vi "Real Time Tracking System of a Colored object.vi"(0 "ROI Descriptor (Color Location 1)":T2={"Global Rectangle"=[20, 20, 1260, 700], "Contours"=[{"ID"=enum."External", "Type"=12, "Coordinates"=[20, 20, 1260, 700, 0]}]} {"Contours"."Type" items=["No Selection", "Point", "Line", "Rectangle", "Oval", "Polygon", "Freehand Region", "Annulus", "Unused2", "Unused3", "Broken Line", "Freehand Line", "Rotated Rectangle"]}, 1 "File Path (Color Location 1)":path=path "E:/engineering courses/my/Machine Vision LV/T.png", 2 "Minimum Match Score (Color Location 1)":sgl=800.0) -> (20 "Matches (Color Location 1)":T3(array[cluster]) {"Bounding Box"."y" format="%.2f"; "Bounding Box"."x" format="%.2f"; "Position"."y" format="%.2f"; "Position"."x" format="%.2f"; "Score" format="%.2f"; "Scale" format="%.2f"; "Angle" format="%.2f"}, 21 "Matches (calibrated) (Color Location 1)":T3(array[cluster]) {"Bounding Box"."y" format="%.2f"; "Bounding Box"."x" format="%.2f"; "Position"."y" format="%.2f"; "Position"."x" format="%.2f"; "Score" format="%.2f"; "Scale" format="%.2f"; "Angle" format="%.2f"}, 22 "Number of Matches (Color Location 1)":i32, 27 "error out":errorcluster)   [LabVIEW 2015]
uses:
  <vilib>/vision/NI_Vision_Development_Module.lvlib
  <resource>/objmgr/imaqdx.rc
  <vilib>/vision/driver/NI_Vision_Acquisition_Software.lvlib
panel:
  out "Image":T1(plugin-control)
  in  "Camera Name":refnum<k21> caption="IMAQdx Session"
  in  "Video Modes":i32(listbox)
  in  "Stop":bool
  out "Buffer Number":u32
  out "Frame Rate":dbl(knob) scale=0.0..100.0
  out "Image Out":T1(plugin-control)
  # "Machine vision application Developed \nBy Abdalrahman M. Amer \nMUST university @Egypt \nabdalrahman.m5959@gmail.com"
  # "Colored Object Tracking system"
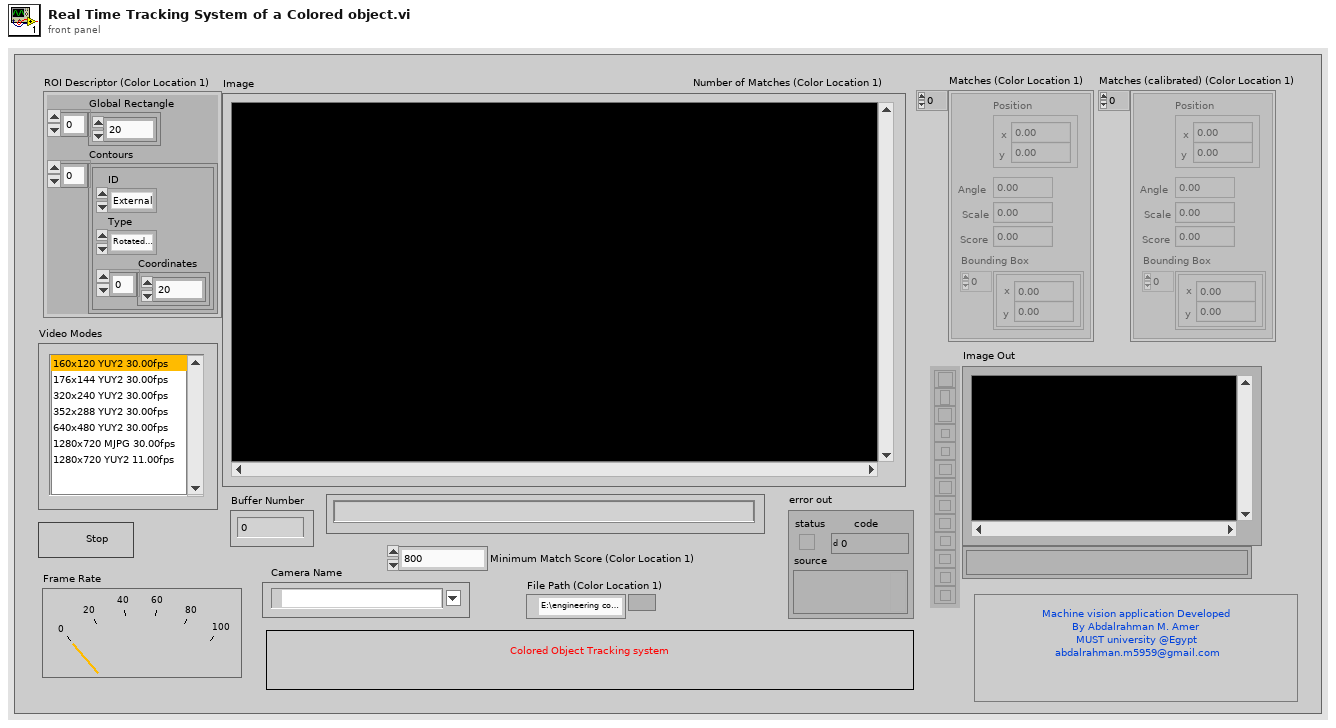
[diagram p1: front panel]
types:
  T1 = typedef "IMAQ Image.ctl" = refnum<image>
  T2 = cluster{"Global Rectangle":i32[], "Contours":cluster{"ID":enum32{"External", "Internal"}, "Type":u32, "Coordinates":i32[]}[]}
  T3 = cluster{"Position":cluster{"x":sgl, "y":sgl}, "Angle":sgl, "Scale":sgl, "Score":sgl, "Bounding Box":cluster{"x":sgl, "y":sgl}[]}[]
  T4 = typedef "IMAQdx.ctl" = refnum<k21>
  T5 = typedef "Image Type" = u32
  T6 = cluster{"Matches[0]":cluster{"Position":cluster{"x":sgl, "y":sgl}, "Angle":sgl, "Scale":sgl, "Score":sgl, "Bounding Box":cluster{"x":sgl, "y":sgl}[]}, "Matches[1]":cluster{"Position":cluster{"x":sgl, "y":sgl}, "Angle":sgl, "Scale":sgl, "Score":sgl, "Bounding Box":cluster{"x":sgl, "y":sgl}[]}, "Matches[2]":cluster{"Position":cluster{"x":sgl, "y":sgl}, "Angle":sgl, "Scale":sgl, "Score":sgl, "Bounding Box":cluster{"x":sgl, "y":sgl}[]}, "Matches[3]":cluster{"Position":cluster{"x":sgl, "y":sgl}, "Angle":sgl, "Scale":sgl, "Score":sgl, "Bounding Box":cluster{"x":sgl, "y":sgl}[]}, "Matches[4]":cluster{"Position":cluster{"x":sgl, "y":sgl}, "Angle":sgl, "Scale":sgl, "Score":sgl, "Bounding Box":cluster{"x":sgl, "y":sgl}[]}, "Matches[5]":cluster{"Position":cluster{"x":sgl, "y":sgl}, "Angle":sgl, "Scale":sgl, "Score":sgl, "Bounding Box":cluster{"x":sgl, "y":sgl}[]}, "Matches[6]":cluster{"Position":cluster{"x":sgl, "y":sgl}, "Angle":sgl, "Scale":sgl, "Score":sgl, "Bounding Box":cluster{"x":sgl, "y":sgl}[]}, "Matches[7]":cluster{"Position":cluster{"x":sgl, "y":sgl}, "Angle":sgl, "Scale":sgl, "Score":sgl, "Bounding Box":cluster{"x":sgl, "y":sgl}[]}, "Matches[8]":cluster{"Position":cluster{"x":sgl, "y":sgl}, "Angle":sgl, "Scale":sgl, "Score":sgl, "Bounding Box":cluster{"x":sgl, "y":sgl}[]}}
  T7 = cluster{"Position":cluster{"x":sgl, "y":sgl}, "Angle":sgl, "Scale":sgl, "Score":sgl, "Bounding Box":cluster{"x":sgl, "y":sgl}[]}
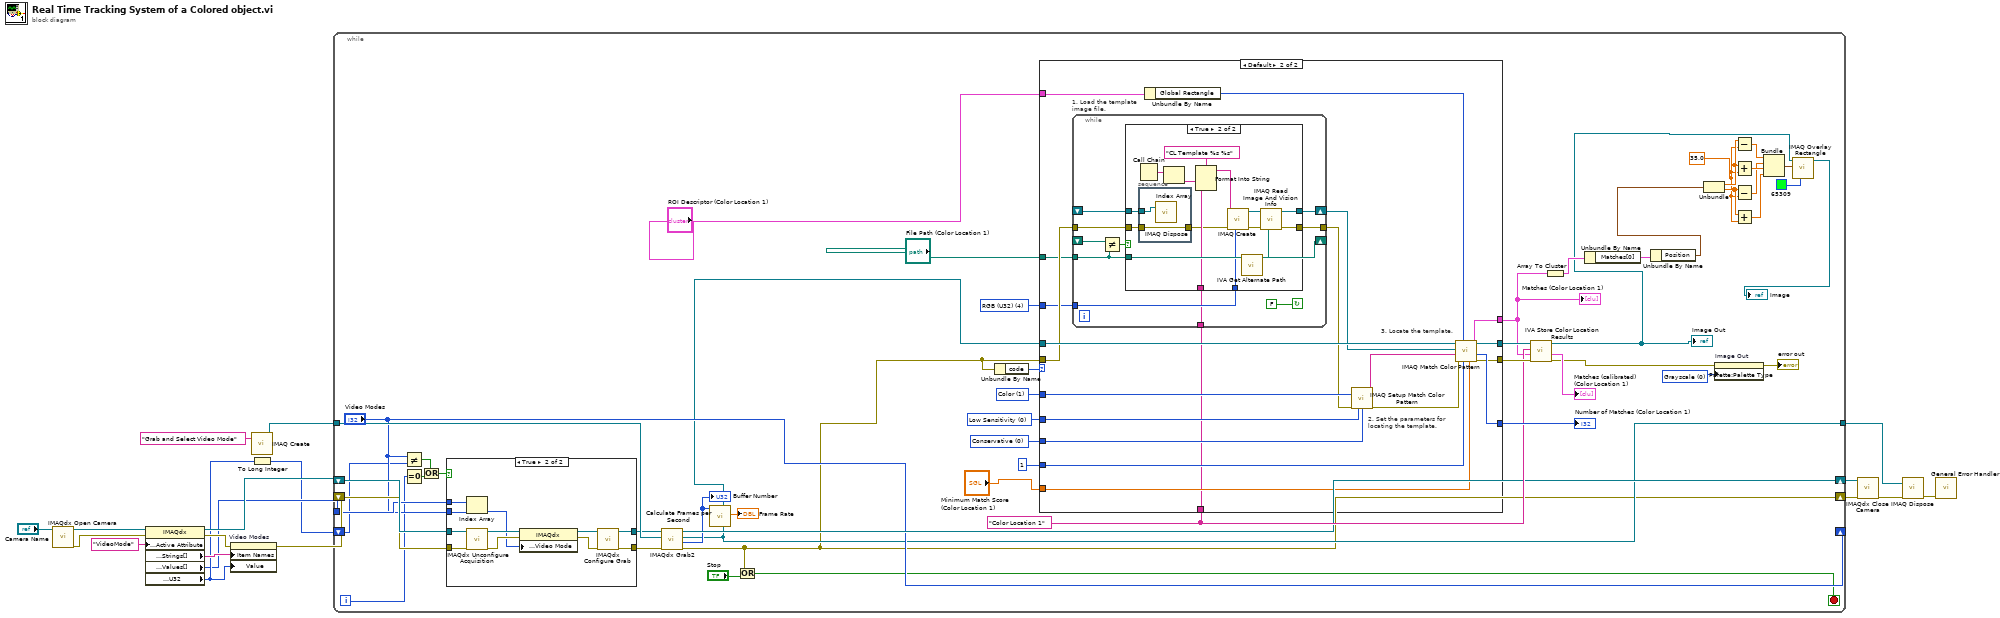
[diagram p0: block diagram]
diagram:
  n1 = call <vilib>:"IMAQdx Open Camera.vi"("Session In"="Camera Name") -> ("error out"=w11:errorcluster, "Session Out"=w13:T4)  [unwired: 2 in, 7 out]
  n2 = property class="IMAQdx"(reference=w13, error in=w11, "Camera Attributes:Active Attribute"="VideoMode" ("ActiveAttribute")) -> (reference out=w9:T4, error out=w10:errorcluster, "Camera Attributes:Enum:Strings[]"=w7:string[], "Camera Attributes:Enum:Values[]"=w2:u32[], "Camera Attributes:Value:U32"=w6:u32)
  n3 = property on="Video Modes" class="LstBox (strict)"(error in=w10, "Item Names"=w7, "Value"=w6) -> (error out=w8:errorcluster)  [unwired: 1 in, 1 out]
  n4 = call "IMAQ Create"("Image Name"="Grab and Select Video Mode") -> ("New Image"=w16:T1)  [unwired: 3 in, 2 out]
  n5 = To Long Integer(number=w6) -> (32bit integer=w1:i32)
  n6 = while {
    tunnel: w2 -> [w48]
    shift-right: [w51] -> w15
    shift-left: w9 -> [w50]
    shift-right: [w34] -> w18
    shift-left: w8 -> [w49]
    tunnel: w16 -> [w52]
    tunnel: [w35] -> w5
    shift-right: ["Video Modes"] -> _
    shift-left: w1 -> [w38]
    i -> [w36]
    stop <- w37 stop-if-true
    w20 = 35.0
    w53 = u32 0 items=["Grayscale", "Binary", "Gradient", "Rainbow", "Temperature", "User Defined", "Binary 16 Bit", "Gradient 16 Bit", "Rainbow 16 Bit", "Temperature 16 Bit", "User Defined 16 Bit"] ("Palette Type")
    w55 = "Color Location 1" ("Step Name")
    w62 = T5 4 items=["Grayscale (U8)", "Grayscale (I16)", "Grayscale (SGL)", "Complex (CSG)", "RGB (U32)", "HSL (U32)", "RGB (U64)"] ("Image Type")
    w64 = u32 0 items=["Conservative", "Balance", "Aggressive", "Very Aggressive"] ("Search Strategy")
    w65 = u32 0 items=["Low Sensitivity", "Medium Sensitivity", "High Sensitivity"] ("Color Sensitivity")
    w66 = u32 1 items=["Color and Shape", "Color", "Shape"] ("Match Feature Mode")
    n7 = Not Equal?(x="Video Modes", y=w38) -> (x != y?=w45:bool)
    n8 = Equal To 0?(x=w36) -> (x = 0?=w44:bool)
    n9 = Or(x=w45, y=w44) -> (x .or. y?=w46:bool)
    n10 = case shown="True" w46 {
      tunnel: w50 -> [w71 w80]
      tunnel: w49 -> [w70 w79]
      tunnel: [w71 w76] -> w42
      tunnel: [w70 w77] -> w43
      tunnel: w48 -> [_ w82]
      tunnel: "Video Modes" -> [_ w81]
      frame False {
      }
      frame True {
        n11 = Index Array(array=w82, index=w81) -> (element=w72:u32)
        n12 = call <vilib>:"IMAQdx Unconfigure Acquisition.vi"("error in"=w79, "Session In"=w80) -> ("error out"=w73:errorcluster, "Session Out"=w78:T4)  [unwired: 8 out]
        n13 = property class="IMAQdx"(reference=w78, error in=w73, "Acquisition Attributes:Video Mode"=w72) -> (reference out=w75:T4, error out=w74:errorcluster)
        n14 = call <vilib>:"IMAQdx Configure Grab.vi"("error in"=w74, "Session In"=w75) -> ("error out"=w77:errorcluster, "Session Out"=w76:T4)  [unwired: 1 in, 7 out]
      }
    }
    n15 = call <vilib>:"IMAQdx Grab2.vi"("error in"=w43, "Image In"=w52, "Session In"=w42) -> ("error out"=w34:errorcluster, "Buffer Number Out"=w40:u32, "Image Out"=w35:T1, "Session Out"=w51:T4)  [unwired: 5 in]
    "Buffer Number" <- w40
    n16 = call <vilib>:"Calculate Frames per Second.vi"("Buffer Number"=w40) -> ("Processed Frames/s"=→"Frame Rate":dbl)  [unwired: 8 in, 2 out]
    n17 = Or(x=w34, y="Stop") -> (x .or. y?=w37:bool)
    n18 = Unbundle By Name(w34) -> ("code"=w60:i32)
    n19 = case shown="Default" w60 {
      tunnel: "Minimum Match Score (Color Location 1)" -> [_ w102]
      tunnel: 1 ("Number of Matches Requested") -> [_ w101]
      tunnel: [_ w100] -> w67
      tunnel: w66 -> [_ w99]
      tunnel: w65 -> [_ w98]
      tunnel: w64 -> [_ w97]
      tunnel: "File Path (Color Location 1)" -> [_ w90]
      tunnel: w62 -> [_ w89]
      tunnel: w34 -> [_ w91]
      tunnel: "ROI Descriptor (Color Location 1)" -> [_ w94]
      tunnel: [_ w84] -> w33
      tunnel: w35 -> [w83 w92]
      tunnel: [w83 w92] -> w56
      tunnel: [_ w86] -> w57
      tunnel: w55 -> [_ w85]
      frame -1074396199, -1074396198 {
        # "Discard Coordinate System Error"
      }
      frame Default {
        # "3. Locate the template."
        # "2. Set the parameters for\nlocating the template."
        n20 = while "1. Load the template image file." {
          shift-right: [w112] -> w88
          shift-left: _ -> [w111]
          tunnel: [w109] -> w87
          tunnel: w91 -> [w108]
          tunnel: w90 -> [w103]
          tunnel: w89 -> [w107]
          tunnel: w85 -> [w106]
          shift-right: [w103] -> _
          shift-left: _ -> [w105]
          stop <- FALSE continue-if-true
          n21 = Not Equal?(x=w105, y=w103) -> (x != y?=w104:bool)
          n22 = case shown="True" w104 {
            tunnel: [w114 w127] -> w112
            tunnel: w111 -> [w114 w119]
            tunnel: [w113 w124] -> w109
            tunnel: w108 -> [w113 w118]
            tunnel: w107 -> [_ w123]
            tunnel: w106 -> [_ w120]
            tunnel: w103 -> [_ w116]
            frame False {
            }
            frame True {
              n23 = Call Chain() -> (call chain=w122:string[])
              n24 = stacked-sequence {
                tunnel: w119 -> [w131]
                tunnel: w118 -> [w130]
                tunnel: [w130] -> w117
                frame #0 {
                  n25 = call "IMAQ Dispose"("Image"=w131) -> ()  [unwired: 2 in, 4 out]
                }
              }
              n26 = Index Array(array=w122) -> (element=w121:string)  [unwired: 1 in]
              n27 = Format Into String(format string="CL Template %s %s" ("Image Name"), w121, w120) -> (resulting string=w129:string)  [unwired: 2 in, 1 out]
              n28 = call "IMAQ Create"("Image Name"=w129, "Image Type"=w123, "error in (no error)"=w117) -> ("New Image"=w126:T1, "error out"=w125:errorcluster)  [unwired: 1 in, 1 out]
              n29 = call <vilib>:"IVA Get Alternate Path.vi"("Path In"=w116) -> ("Path Out"=w115:path)  [unwired: 10 out]
              n30 = call "IMAQ Read Image And Vision Info"("File Path"=w115, "error in (no error)"=w125, "Image"=w126) -> ("error out"=w124:errorcluster, "Image Out"=w127:T1)  [unwired: 1 in, 6 out]
            }
          }
        }
        n31 = Unbundle By Name(w94) -> ("Global Rectangle"=w93:i32[])
        n32 = call "IMAQ Setup Match Color Pattern"("Match Feature Mode"=w99, "error in (no error)"=w87, "Color Sensitivity"=w98, "Search Strategy"=w97) -> ("Match Color Pattern Setup Data"=w96:string, "error out"=w95:errorcluster)  [unwired: 5 in, 5 out]
        n33 = call "IMAQ Match Color Pattern"("Minimum Match Score"=w102, "Number of Matches Requested"=w101, "Optional Rectangle"=w93, "error in (no error)"=w95, "Match Color Pattern Setup Data"=w96, "Template Image"=w88, "Image"=w92) -> ("error out"=w86:errorcluster, "Number of Matches"=w100:i32, "Matches"=w84:T3)  [unwired: 2 out]
      }
    }
    "Number of Matches (Color Location 1)" <- w67
    "Matches (Color Location 1)" <- w33
    n34 = call <vilib>:"IVA Store Color Location Results.vi"("error in (no error)"=w57, "Matches"=w33, "Step Name"=w55, "Image in"=w56) -> ("error out"=w58:errorcluster, "Calibrated Matches"=→"Matches (calibrated) (Color Location 1)":T3, "Image dup"=w29:T1)  [unwired: 5 out]
    "Image Out" <- w29
    n35 = Array To Cluster(array=w33) -> (cluster=w32:T6)
    n36 = Unbundle By Name(w32) -> ("Matches[0]"=w31:T7)
    n37 = Unbundle By Name(w31) -> ("Position"=w30:cluster{"x":sgl, "y":sgl})
    n38 = Unbundle(w30) -> ("x"=w21:sgl, "y"=w24:sgl)
    n39 = property on="Image Out" class="ImageControl"(error in=w58, "Palette:Palette Type"=w53) -> (error out=→"error out":errorcluster)  [unwired: 1 in, 1 out]
    n40 = Subtract(x=w21, y=w20) -> (x-y=w26:dbl)
    n41 = Add(x=w21, y=w20) -> (x+y=w27:dbl)
    n42 = Subtract(x=w24, y=w20) -> (x-y=w23:dbl)
    n43 = Add(x=w24, y=w20) -> (x+y=w25:dbl)
    n44 = Bundle(w26, w23, w27, w25) -> (w22:cluster{dbl, dbl, dbl, dbl})  [unwired: 1 in]
    n45 = call "IMAQ Overlay Rectangle"("Color"=u32 65309, "Rectangle"=w22, "Image"=w29) -> ("Image Out"=→"Image":T1)  [unwired: 7 in, 1 out]
  }
  n46 = call <vilib>:"IMAQdx Close Camera.vi"("error in"=w18, "Session In"=w15) -> ("error out"=w4:errorcluster)  [unwired: 9 out]
  n47 = call "IMAQ Dispose"("Image"=w5, "error in (no error)"=w4) -> ("error out"=w3:errorcluster)  [unwired: 4 in]
  n48 = call <vilib>:"General Error Handler.vi"("error in (no error)"=w3) -> ()  [unwired: 2 in, 13 out]
